vi "Find next available folder name.vi"(11 "Input folder":path=path "C:/Users/Optix/Dropbox (MIT)/Research/Backup/66-225 Optix data/Yiming MO/AC electrolysis/HPLC data backup") -> (3 "Output folder":path=path "C:/Users/Optix/Dropbox (MIT)/Research/Backup/66-225 Optix data/Yiming MO/AC electrolysis/HPLC data backup")   [LabVIEW 2017]
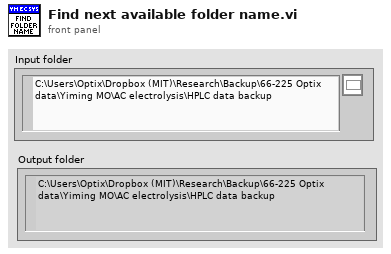
[diagram p1: front panel]
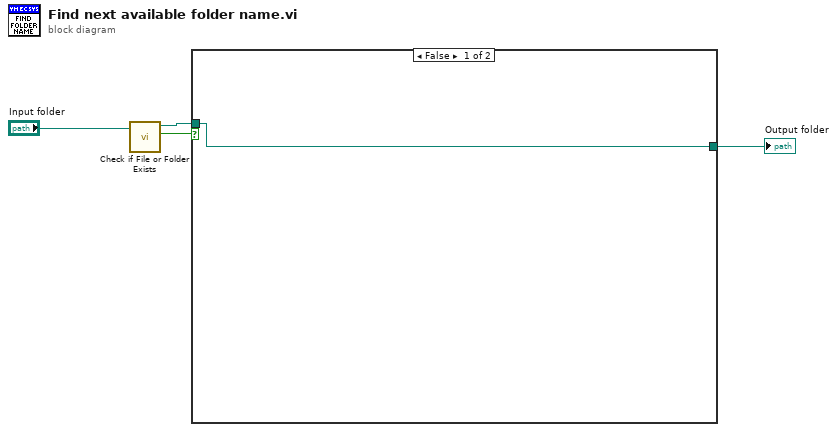
[diagram p0: block diagram]
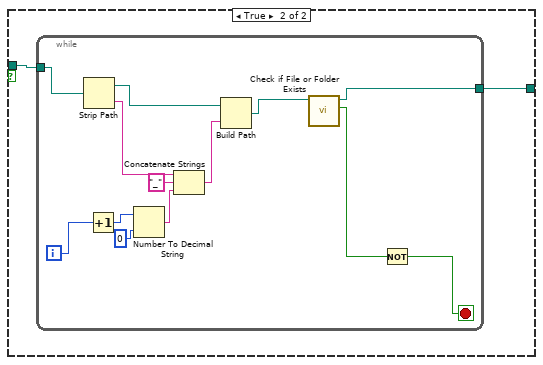
[diagram p2: hidden frame]
diagram:
  n1 = call <vilib>:"Check if File or Folder Exists.vi"("path"="Input folder") -> ("file or folder exists?"=w3:bool, "dup path"=w2:path)  [unwired: 8 in, 1 out]
  n2 = case shown="False" w3 {
    tunnel: w2 -> [w5 w7]
    tunnel: [w5 w6] -> w1
    frame False {
    }
    frame True {
      n3 = while {
        tunnel: w7 -> [w20]
        tunnel: [w8] -> w6
        i -> [w18]
        stop <- w10 stop-if-true
        n4 = Strip Path(path=w20) -> (stripped path=w19:path, name=w14:string)
        n5 = Increment(x=w18) -> (x+1=w17:i32)
        n6 = Number To Decimal String(number=w17, width (-)=i16 0) -> (decimal integer string=w13:string)
        n7 = Concatenate Strings(w14, "_" ("string"), w13) -> (w15:string)
        n8 = Build Path(base path=w19, name or relative path=w15) -> (appended path=w11:path)
        n9 = call <vilib>:"Check if File or Folder Exists.vi"("path"=w11) -> ("file or folder exists?"=w9:bool, "dup path"=w8:path)  [unwired: 8 in, 1 out]
        n10 = Not(x=w9) -> (.not. x?=w10:bool)
      }
    }
  }
  "Output folder" <- w1
